vi "GenerateUniqueName.vi"(10 "Name":string, 11 "ObjectTable":cluster{"Name":string, "ObjectRef":refnum<vi>}[](array[cluster])) -> (3 "UniqueName":string)   [LabVIEW 2014]
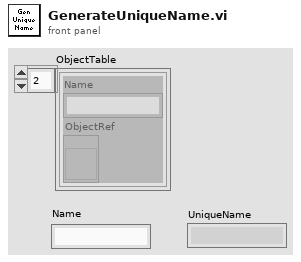
[diagram p1: front panel]
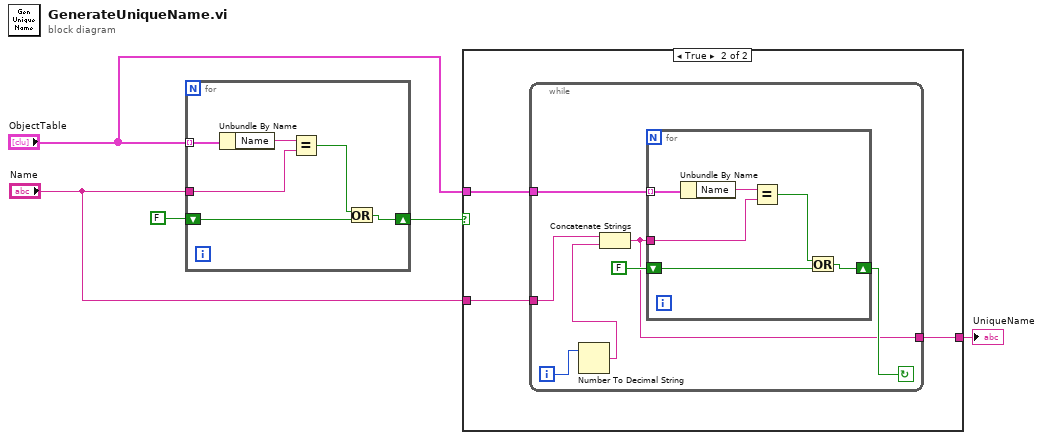
[diagram p0: block diagram]
diagram:
  n1 = for {
    tunnel: "ObjectTable" -> [w11] mode=indexing
    tunnel: "Name" -> [w9]
    shift-right: [w7] -> w4
    shift-left: FALSE -> [w8]
    n2 = Unbundle By Name(w11) -> ("Name"=w10:string)
    n3 = Equal?(x=w10, y=w9) -> (x = y?=w6:bool)
    n4 = Or(x=w6, y=w8) -> (x .or. y?=w7:bool)
  }
  n5 = case shown="True" w4 {
    tunnel: "ObjectTable" -> [_ w15]
    tunnel: "Name" -> [w12 w14]
    tunnel: [w12 w13] -> w1
    frame False {
    }
    frame True {
      n6 = while {
        tunnel: w15 -> [w21]
        tunnel: w14 -> [w17]
        tunnel: [w16] -> w13
        i -> [w20]
        stop <- w19 continue-if-true
        n7 = Number To Decimal String(number=w20) -> (decimal integer string=w18:string)  [unwired: 1 in]
        n8 = Concatenate Strings(w17, w18) -> (w16:string)
        n9 = for {
          tunnel: w21 -> [w28] mode=indexing
          tunnel: w16 -> [w26]
          shift-right: [w24] -> w19
          shift-left: FALSE -> [w25]
          n10 = Unbundle By Name(w28) -> ("Name"=w27:string)
          n11 = Equal?(x=w27, y=w26) -> (x = y?=w23:bool)
          n12 = Or(x=w23, y=w25) -> (x .or. y?=w24:bool)
        }
      }
    }
  }
  "UniqueName" <- w1
